vi "Servo.vi"() -> ()   [LabVIEW 2024]
uses:
  Driver/CTIPicoVISA.lvlib
panel:
  in  "Freq Hz":sgl=600.0
  in  "Degrees":u16(slide) scale=0.0..360.0
  out "Identity":T1
  in  "GroveConnector":enum16{"A0", "A1", "A2"}(ring)
  in  "stop":bool
  in  "VISA resource name in":refnum<visa-resource-name>="COM7"
  out "error out":errorcluster
  # "https://wiki.seeedstudio.com/Grove-Servo/"
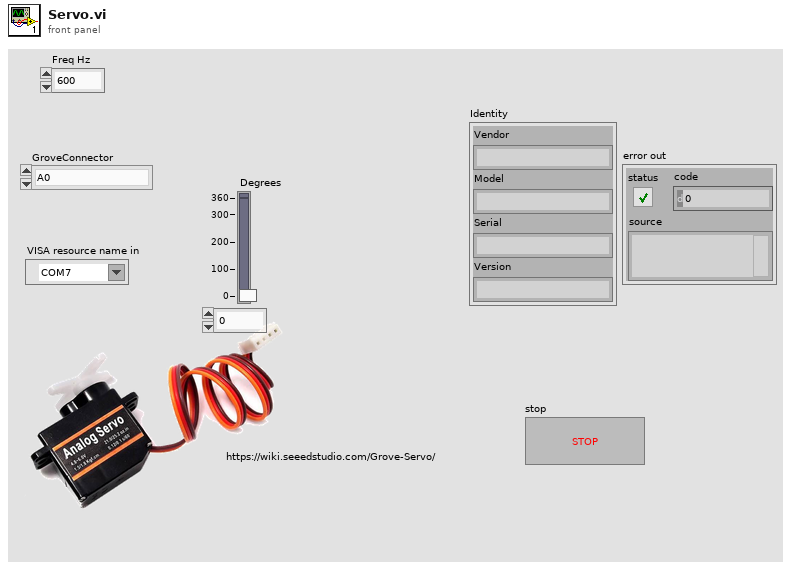
[diagram p1: front panel]
types:
  T1 = cluster{"Vendor":string, "Model":string, "Serial":string, "Version":string}
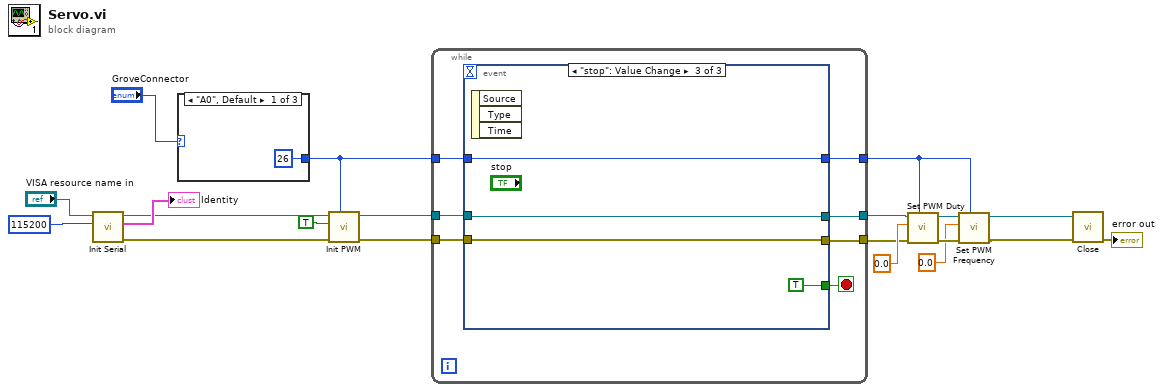
[diagram p0: block diagram]
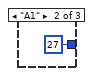
[diagram p2: hidden frame]
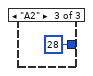
[diagram p3: hidden frame]
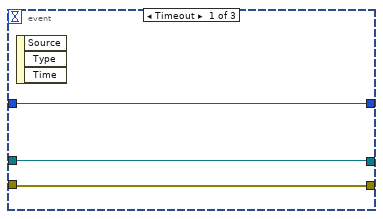
[diagram p4: hidden frame]
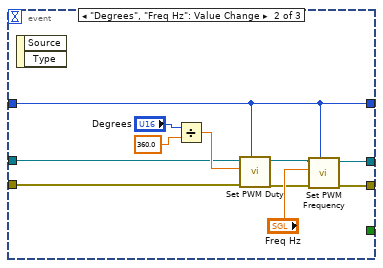
[diagram p5: hidden frame]
diagram:
  n1 = call "Init Serial.vi"("Baud (115200)"=u32 115200, "VISA resource name in"="VISA resource name in") -> ("error out"=w14:errorcluster, "Identity"=→"Identity":T1, "VISA resource name Out"=w15:refnum<visa-resource-name>)  [unwired: 7 in]
  n2 = case shown="\"A0\", Default" "GroveConnector" {
    tunnel: [26 ("GPIO") 27 ("GPIO") 28 ("GPIO")] -> w5
    frame "A0", Default {
    }
    frame "A1" {
    }
    frame "A2" {
    }
  }
  n3 = call "Init PWM.vi"("GPIO"=w5, "error in (no error)"=w14, "Enable (F)"=TRUE, "VISA resource name in"=w15) -> ("error out"=w2:errorcluster, "VISA resource name"=w1:refnum<visa-resource-name>)  [unwired: 6 in]
  n4 = while {
    tunnel: w1 -> [w29]
    tunnel: w5 -> [w28]
    tunnel: w2 -> [w30]
    tunnel: [w26] -> w7
    tunnel: [w27] -> w8
    tunnel: [w25] -> w6
    stop <- w24 stop-if-true
    n5 = event shown="[2] \"stop\": Value Change" {
      selector: _ -> [_ _ _]
      dyn-events: _ -> [_ _ _]
      timeout: _ -> [_ _ _]
      tunnel: w30 -> [w31 w37 w46]
      tunnel: w29 -> [w32 w38 w47]
      tunnel: w28 -> [w33 w34 w48]
      tunnel: [w32 w36 w47] -> w27
      tunnel: [w31 w35 w46] -> w26
      tunnel: [w33 w34 w48] -> w25
      tunnel: [_ _ TRUE] -> w24
      event Timeout {
        n6 = event-data() -> ()  [unwired: 1 in, 3 out]
      }
      event "Degrees", "Freq Hz": Value Change {
        n7 = event-data() -> ()  [unwired: 1 in, 2 out]
        n8 = Divide(x="Degrees", y=sgl 360.0 ("Freq Hz")) -> (x/y=w43:sgl)
        n9 = call "Set PWM Duty.vi"("GPIO"=w34, "error in (no error)"=w37, "Duty % (0-1)"=w43, "VISA resource name in"=w38) -> ("error out"=w40:errorcluster, "VISA resource name"=w41:refnum<visa-resource-name>)  [unwired: 6 in]
        n10 = call "Set PWM Frequency.vi"("GPIO"=w34, "error in (no error)"=w40, "Freq Hz"="Freq Hz", "VISA resource name in"=w41) -> ("error out"=w35:errorcluster, "VISA resource name"=w36:refnum<visa-resource-name>)  [unwired: 6 in]
      }
      event "stop": Value Change {
        n11 = event-data() -> ()  [unwired: 1 in, 3 out]
      }
    }
  }
  n12 = call "Set PWM Duty.vi"("GPIO"=w6, "error in (no error)"=w7, "Duty % (0-1)"=sgl 0.0, "VISA resource name in"=w8) -> ("error out"=w12:errorcluster, "VISA resource name"=w11:refnum<visa-resource-name>)  [unwired: 6 in]
  n13 = call "Set PWM Frequency.vi"("GPIO"=w6, "error in (no error)"=w12, "Freq Hz"=sgl 0.0, "VISA resource name in"=w11) -> ("error out"=w3:errorcluster, "VISA resource name"=w4:refnum<visa-resource-name>)  [unwired: 6 in]
  n14 = call "Close.vi"("error in (no error)"=w3, "VISA resource name in"=w4) -> ("error out"=→"error out":errorcluster)  [unwired: 9 in]
